vi "Save System errors.vi"(11 "Error Text":string) -> ()   [LabVIEW 2023]
uses:
  <vilib>/Utility/file.llb/Write Delimited Spreadsheet (string).vi
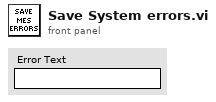
[diagram p1: front panel]
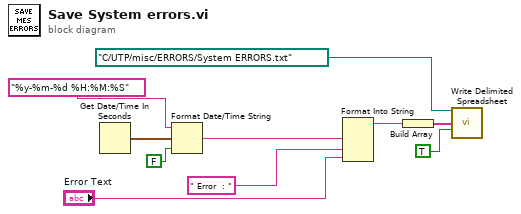
[diagram p0: block diagram]
diagram:
  n1 = Get Date/Time In Seconds() -> (seconds since 1Jan1904=w7:timestamp)
  n2 = Format Date/Time String(time format string (%c)="%y-%m-%d %H:%M:%S", seconds (now)=w7, UTC format=FALSE) -> (date/time string=w4:string)
  n3 = Format Into String(w4, " Error  : " ("input 2"), "Error Text") -> (resulting string=w2:string)  [unwired: 3 in, 1 out]
  n4 = Build Array(w2) -> (w8:string[])
  n5 = call-poly <vilib>:"Write Delimited Spreadsheet.vi"("file path (dialog if empty)"=path "C:/UTP/misc/ERRORS/System ERRORS.txt", "1D data"=w8, "append to file? (new file:F)"=TRUE) -> ()  [unwired: 11 in, 2 out]
